vi "AEROTECstageAPIgfv.vi"(8 "error in (no error)":errorcluster, 10 "Data in":variant, 11 "StageContrlEnum":T1=enum."Init") -> (0 "error out":errorcluster, 3 "Data Out":variant)   [LabVIEW 2017]
doc: "Use this template to build a VI to use as a subVI."
uses:
  StageEnum.ctl
  MoveDistanceInAxis.ctl
  Utility/AxisControl.ctl
  SingleStageData.ctl
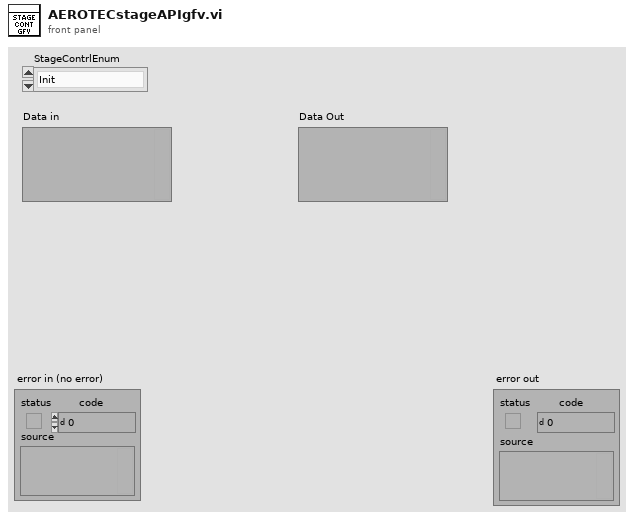
[diagram p1: front panel]
types:
  T1 = typedef "StageEnum.ctl" = enum16{"Get Current Pos!", "Move axis!", "Enable Stage!", "Stop Stage Controller!", "Set Default Speeds!", "Get Stage Parameters", "Start Stage Controller!", "Init", "Go Home!"}
  T2 = typedef "AxisControl.ctl" = cluster{"Axis":string, "Enable":bool, "Disable":bool, "Home":bool, "FaultAck":bool, "Jog":bool, "Speed":dbl, "Distance":dbl, "Jog Left":bool, "Jog Right":bool, "Status":string, "Pos Fbk":dbl, "Vel Fbk":dbl, "Pos Units":string, "Vel Units":string}
  T3 = enum32{"Invalid", "Standard", "Closed", "Hidden", "Minimized", "Maximized"}
  T4 = typedef "SingleStageData.ctl" = cluster{"Desired Speed(mm/s)":dbl, "Desired Distance(mm)":dbl, "Enabled?":bool, "Moving?":bool, "Position(microns)":dbl}
  T5 = typedef "MoveDistanceInAxis.ctl" = cluster{"Axis Number":i16, "Distance (microns)":dbl}
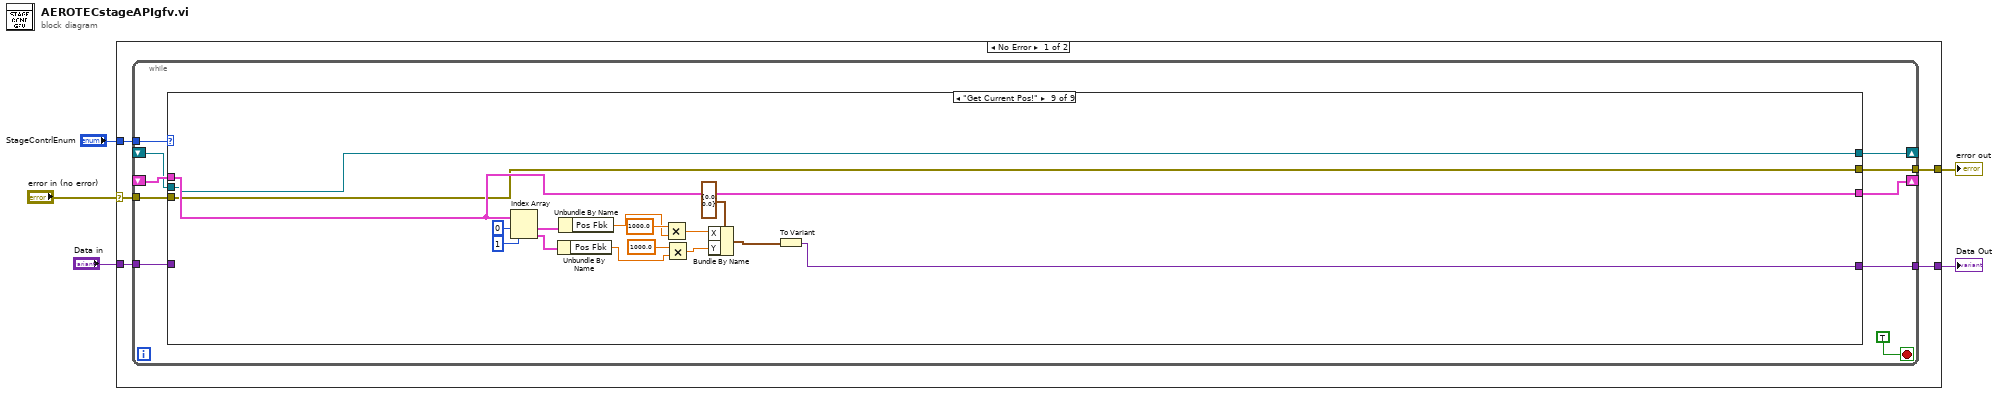
[diagram p0: block diagram]
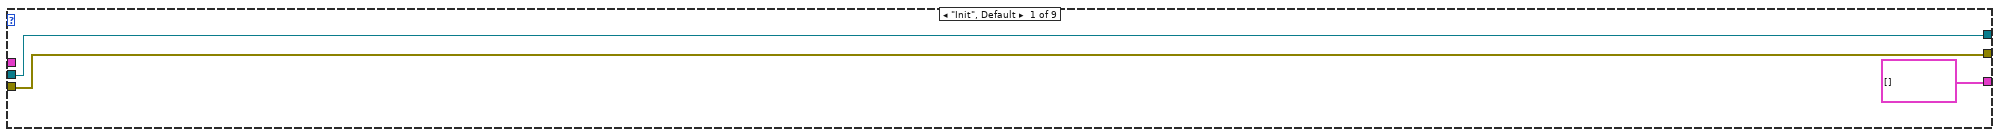
[diagram p2: hidden frame]
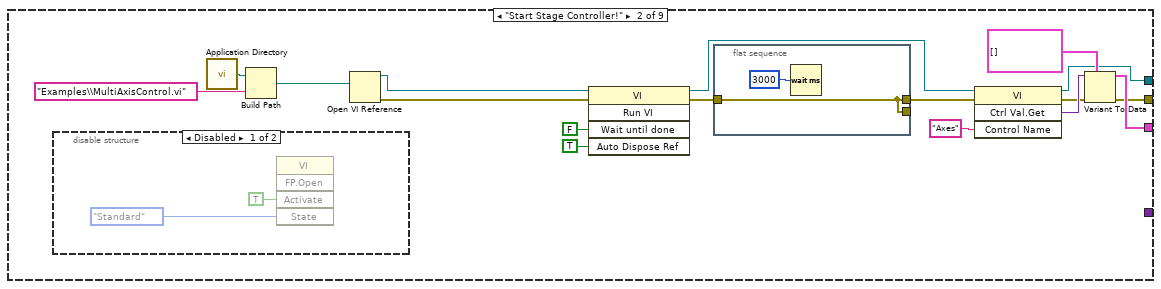
[diagram p3: hidden frame]
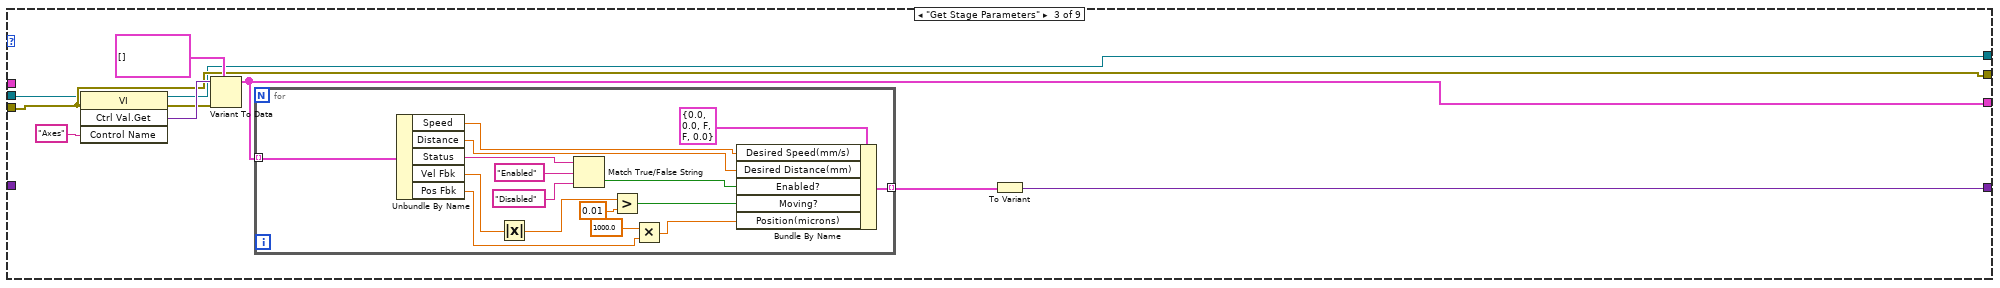
[diagram p5: hidden frame]
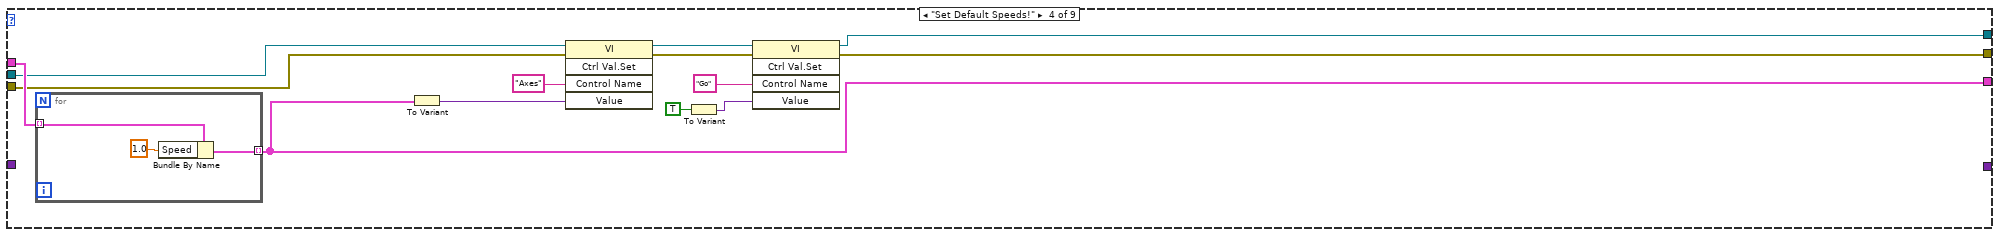
[diagram p6: hidden frame]
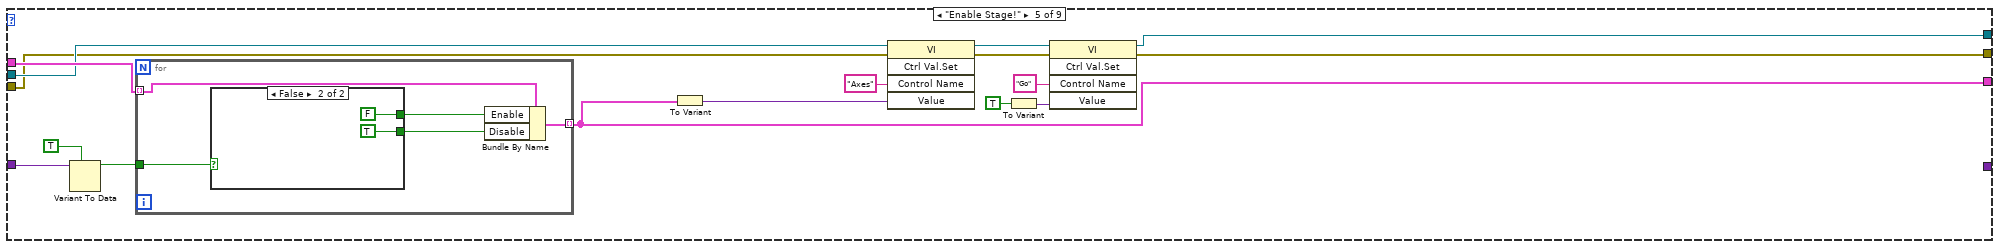
[diagram p7: hidden frame]
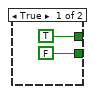
[diagram p8: hidden frame]
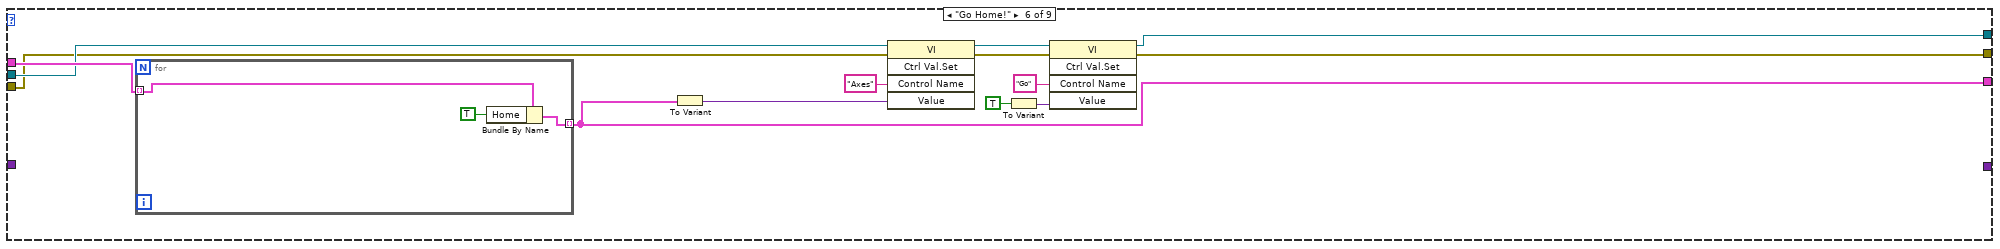
[diagram p9: hidden frame]
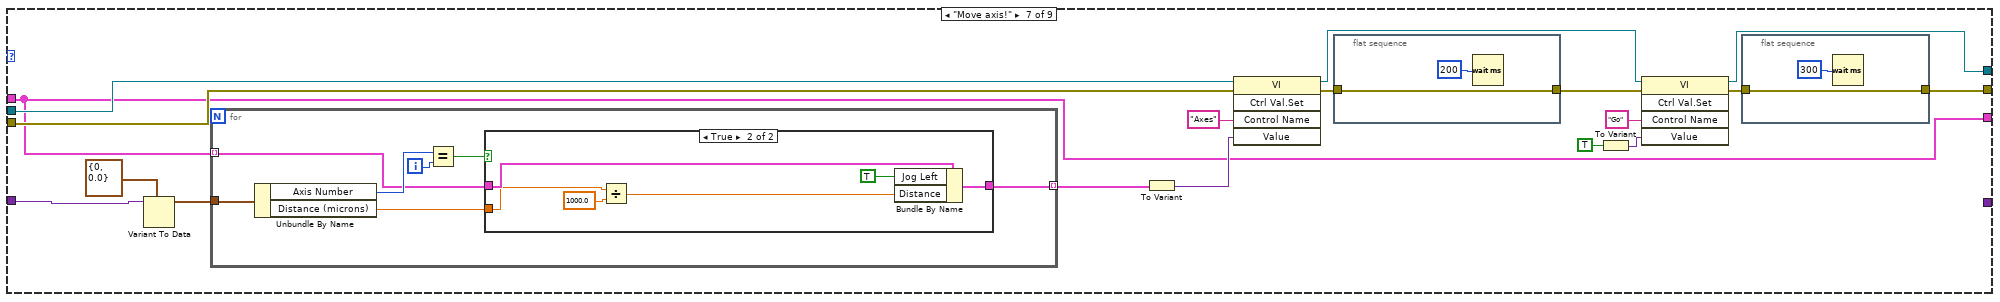
[diagram p10: hidden frame]
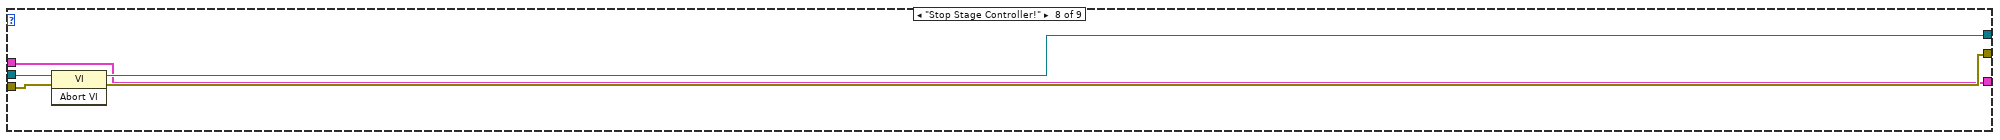
[diagram p12: hidden frame]
diagram:
  n1 = case shown="No Error" "error in (no error)" {
    selector: "error in (no error)" -> [w9 w185]
    tunnel: [w7 w185] -> w4
    tunnel: "Data in" -> [w10 _]
    tunnel: "StageContrlEnum" -> [w8 _]
    tunnel: [w6 _] -> w1
    frame No Error {
      n2 = while {
        tunnel: w10 -> [w19]
        tunnel: w9 -> [w18]
        tunnel: w8 -> [w17]
        shift-right: [w16] -> _
        shift-left: _ -> [w14]
        tunnel: [w15] -> w7
        shift-right: [w13] -> _
        shift-left: _ -> [w12]
        tunnel: [w11] -> w6
        stop <- TRUE stop-if-true
        n3 = case shown="\"Get Current Pos!\"" w17 {
          tunnel: w19 -> [_ _ _ _ w89 _ w137 _ _]
          tunnel: w18 -> [w23 _ w49 w78 w97 w119 w142 w167 w182]
          tunnel: [T2[] [] w31 w46 w79 w98 w120 w133 w164 w184] -> w16
          tunnel: [w23 w30 w49 w72 w90 w112 w128 w166 w182] -> w15
          tunnel: w14 -> [_ _ _ w83 w102 w124 w133 w164 w184]
          tunnel: [w21 w28 w47 w73 w91 w113 w132 w165 w183] -> w13
          tunnel: w12 -> [w21 _ w48 w80 w99 w121 w143 w168 w183]
          tunnel: [_ _ w53 _ _ _ _ _ w175] -> w11
          frame "Init", Default {
          }
          frame "Start Stage Controller!" {
            n4 = disable-structure shown="Disabled" {
              frame Disabled {
                n5 = invoke class="VI" method="FP.Open"("Activate"=TRUE ("Wait Until Done"), "State"=T3."Standard") -> ()  [unwired: 3 in, 5 out]
              }
              frame Enabled {
              }
            }
            n6 = call <vilib>:"Application Directory.vi"() -> ("Application Directory"=w38:path)
            n7 = Build Path(base path=w38, name or relative path="Examples\\MultiAxisControl.vi") -> (appended path=w36:path)
            n8 = Open VI Reference(vi path=w36) -> (vi reference=w25:refnum<vi>, error out=w24:errorcluster)  [unwired: 5 in]
            n9 = invoke class="VI" method="Run VI"(reference=w25, error in=w24, "Wait until done"=FALSE ("Wait Until Done"), "Auto Dispose Ref"=TRUE ("Auto Dispose Reference")) -> (reference out=w32:refnum<vi>, error out=w27:errorcluster)  [unwired: 1 in, 3 out]
            n10 = flat-sequence {
              tunnel: w27 -> [w43]
              tunnel: [w43] -> _
              tunnel: [w43] -> w26
              frame #0 {
                n11 = Wait (ms)(milliseconds to wait=u32 3000) -> ()  [unwired: 1 out]
              }
            }
            n12 = invoke class="VI" method="Ctrl Val.Get"(reference=w32, error in=w26, "Control Name"="Axes") -> (reference out=w28:refnum<vi>, error out=w29:errorcluster, "Get Control Value Variant"=w34:variant)  [unwired: 1 in, 1 out]
            n13 = Variant To Data(error in=w29, type=T2[] [], Variant=w34) -> (data=w31:T2[], error out=w30:errorcluster)
          }
          frame "Get Stage Parameters" {
            n14 = invoke class="VI" method="Ctrl Val.Get"(reference=w48, error in=w49, "Control Name"="Axes") -> (reference out=w47:refnum<vi>, error out=w50:errorcluster, "Get Control Value Variant"=w51:variant)  [unwired: 1 in, 1 out]
            n15 = Variant To Data(error in=w50, type=T2[] [], Variant=w51) -> (data=w46:T2[])  [unwired: 1 out]
            n16 = for {
              tunnel: w46 -> [w69] mode=indexing
              tunnel: [w58] -> w54 mode=indexing
              n17 = Unbundle By Name(w69) -> ("Speed"=w68:dbl, "Distance"=w67:dbl, "Status"=w66:string, "Vel Fbk"=w61:dbl, "Pos Fbk"=w57:dbl)
              n18 = Absolute Value(x=w61) -> (abs(x)=w62:dbl)
              n19 = Match True/False String(2:"Disabled" ("false string"), 3:"Enabled" ("true string"), 4:w66) -> (0:w63:bool)  [unwired: 1 out]
              n20 = Greater?(x=w62, y=0.01) -> (0:w59:bool)
              n21 = Multiply(x=1000.0, y=w57) -> (x*y=w55:dbl)
              n22 = Bundle By Name(cluster=T4 {"Desired Speed(mm/s)"=0.0, "Desired Distance(mm)"=0.0, "Enabled?"=FALSE, "Moving?"=FALSE, "Position(microns)"=0.0} ("StageParamters"), "Desired Speed(mm/s)"=w68, "Desired Distance(mm)"=w67, "Enabled?"=w63, "Moving?"=w59, "Position(microns)"=w55) -> (w58:T4)
            }
            n23 = To Variant(anything=w54) -> (Variant=w53:variant)
          }
          frame "Set Default Speeds!" {
            n24 = for {
              tunnel: w83 -> [w86] mode=indexing
              tunnel: [w84] -> w79 mode=indexing
              n25 = Bundle By Name(cluster=w86, "Speed"=1.0) -> (w84:T2)
            }
            n26 = To Variant(anything=w79) -> (Variant=w81:variant)
            n27 = invoke class="VI" method="Ctrl Val.Set"(reference=w80, error in=w78, "Control Name"="Axes", "Value"=w81) -> (reference out=w75:refnum<vi>, error out=w74:errorcluster)  [unwired: 1 in, 3 out]
            n28 = To Variant(anything=TRUE) -> (Variant=w77:variant)
            n29 = invoke class="VI" method="Ctrl Val.Set"(reference=w75, error in=w74, "Control Name"="Go", "Value"=w77) -> (reference out=w73:refnum<vi>, error out=w72:errorcluster)  [unwired: 1 in, 3 out]
          }
          frame "Enable Stage!" {
            n30 = Variant To Data(type=TRUE, Variant=w89) -> (data=w87:bool)  [unwired: 1 in, 1 out]
            n31 = for {
              tunnel: w102 -> [w107] mode=indexing
              tunnel: [w106] -> w98 mode=indexing
              tunnel: w87 -> [w105]
              n32 = case shown="False" w105 {
                tunnel: [TRUE FALSE] -> w104
                tunnel: [FALSE TRUE] -> w103
                frame True {
                }
                frame False {
                }
              }
              n33 = Bundle By Name(cluster=w107, "Enable"=w104, "Disable"=w103) -> (w106:T2)
            }
            n34 = To Variant(anything=w98) -> (Variant=w100:variant)
            n35 = invoke class="VI" method="Ctrl Val.Set"(reference=w99, error in=w97, "Control Name"="Axes", "Value"=w100) -> (reference out=w93:refnum<vi>, error out=w92:errorcluster)  [unwired: 1 in, 3 out]
            n36 = To Variant(anything=TRUE) -> (Variant=w95:variant)
            n37 = invoke class="VI" method="Ctrl Val.Set"(reference=w93, error in=w92, "Control Name"="Go", "Value"=w95) -> (reference out=w91:refnum<vi>, error out=w90:errorcluster)  [unwired: 1 in, 3 out]
          }
          frame "Go Home!" {
            n38 = for {
              tunnel: w124 -> [w127] mode=indexing
              tunnel: [w126] -> w120 mode=indexing
              n39 = Bundle By Name(cluster=w127, "Home"=TRUE) -> (w126:T2)
            }
            n40 = To Variant(anything=w120) -> (Variant=w122:variant)
            n41 = invoke class="VI" method="Ctrl Val.Set"(reference=w121, error in=w119, "Control Name"="Axes", "Value"=w122) -> (reference out=w115:refnum<vi>, error out=w114:errorcluster)  [unwired: 1 in, 3 out]
            n42 = To Variant(anything=TRUE) -> (Variant=w117:variant)
            n43 = invoke class="VI" method="Ctrl Val.Set"(reference=w115, error in=w114, "Control Name"="Go", "Value"=w117) -> (reference out=w113:refnum<vi>, error out=w112:errorcluster)  [unwired: 1 in, 3 out]
          }
          frame "Move axis!" {
            n44 = Variant To Data(type=T5 {"Axis Number"=0, "Distance (microns)"=0.0} ("MoveDistanceInAxis"), Variant=w137) -> (data=w135:T5)  [unwired: 1 in, 1 out]
            n45 = for {
              tunnel: w133 -> [w152] mode=indexing
              tunnel: w135 -> [w156]
              tunnel: [w151] -> w134 mode=indexing
              i -> [w153]
              n46 = Unbundle By Name(w156) -> ("Axis Number"=w154:i16, "Distance (microns)"=w150:dbl)
              n47 = Equal?(x=w154, y=w153) -> (x = y?=w155:bool)
              n48 = case shown="True" w155 {
                tunnel: w152 -> [w157 w163]
                tunnel: [w157 w161] -> w151
                tunnel: w150 -> [_ w160]
                frame False {
                }
                frame True {
                  n49 = Divide(x=w160, y=1000.0) -> (x/y=w158:dbl)
                  n50 = Bundle By Name(cluster=w163, "Jog Left"=TRUE, "Distance"=w158) -> (w161:T2)
                }
              }
            }
            n51 = To Variant(anything=w134) -> (Variant=w144:variant)
            n52 = invoke class="VI" method="Ctrl Val.Set"(reference=w143, error in=w142, "Control Name"="Axes", "Value"=w144) -> (reference out=w138:refnum<vi>, error out=w131:errorcluster)  [unwired: 1 in, 3 out]
            n53 = flat-sequence {
              tunnel: [w148] -> w130
              tunnel: w131 -> [w148]
              frame #0 {
                n54 = Wait (ms)(milliseconds to wait=u32 200) -> ()  [unwired: 1 out]
              }
            }
            n55 = To Variant(anything=TRUE) -> (Variant=w140:variant)
            n56 = invoke class="VI" method="Ctrl Val.Set"(reference=w138, error in=w130, "Control Name"="Go", "Value"=w140) -> (reference out=w132:refnum<vi>, error out=w129:errorcluster)  [unwired: 1 in, 3 out]
            n57 = flat-sequence {
              tunnel: [w146] -> w128
              tunnel: w129 -> [w146]
              frame #0 {
                n58 = Wait (ms)(milliseconds to wait=u32 300) -> ()  [unwired: 1 out]
              }
            }
          }
          frame "Stop Stage Controller!" {
            n59 = invoke class="VI" method="Abort VI"(reference=w168, error in=w167) -> (reference out=w165:refnum<vi>, error out=w166:errorcluster)  [unwired: 1 in, 1 out]
          }
          frame "Get Current Pos!" {
            n60 = Index Array(array=w184, index #1=0 ("index"), index #2=1 ("index")) -> (element #1=w179:T2, element #2=w178:T2)
            n61 = Unbundle By Name(w178) -> ("Pos Fbk"=w169:dbl)
            n62 = Unbundle By Name(w179) -> ("Pos Fbk"=w170:dbl)
            n63 = Multiply(x=1000.0, y=w170) -> (x*y=w173:dbl)
            n64 = Multiply(x=1000.0, y=w169) -> (x*y=w171:dbl)
            n65 = Bundle By Name(cluster=cluster{"X":dbl, "Y":dbl} {"X"=0.0, "Y"=0.0} ("Point Coordinates"), "X"=w173, "Y"=w171) -> (w176:cluster{"X":dbl, "Y":dbl})
            n66 = To Variant(anything=w176) -> (Variant=w175:variant)
          }
        }
      }
    }
    frame Error {
    }
  }
  "error out" <- w4
  "Data Out" <- w1
